vi "SeCrTs-UI Commands_R.vi"(9 "Er":refnum<queue>, 11 "Message Queue":refnum<queue>) -> ()   [LabVIEW 2022 SP3]
doc: "Use this template to build a simple state machine design pattern. Each state executes code and determines which state to transition to."
uses:
  RT Controls/SeCrTs-Message Cluster_R.ctl
  RT Controls/SeCrTs-NS Enum.ctl
  RT Controls/SeCrTs-Data Type Control screen.ctl
  RT Support/SeCrTs-RT_Global_R.vi
  <resource>/objmgr/ni.dex.rc
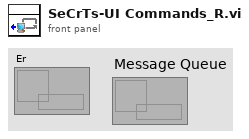
[diagram p1: front panel]
types:
  T1 = typedef "SeCrTs-NS Enum.ctl" = enum16{"Initialize", "Listen for UI Writer", "Receive UI Commands"}
  T2 = typedef "SeCrTs-Data Type Control screen.ctl" = cluster{"DI_Data":digitalwaveform[], "Drive_A_C":waveform(dbl)[], "Drive_A_D":waveform(dbl)[], "Drive_L_C":waveform(dbl)[], "Drive_L_D":waveform(dbl)[], "Loop Status":bool[], "CDT Timer":dbl, "RT Error":cluster{"Error Code":string, "Error Source":string}, "DO":waveform(dbl)[], "SEQ Monitor":string[]}
  T3 = typedef "SeCrTs-Message Cluster_R.ctl" = cluster{"Message":string, "Message Data":variant}
  T4 = typedef "Message Cluster_R.ctl" = cluster{"Message":string, "Message Data":variant}
  T5 = cluster{"Start DAQ":bool, "Stop DAQ":bool, "RT Stop":bool, "RT Exit":bool, "Start Seq":bool}
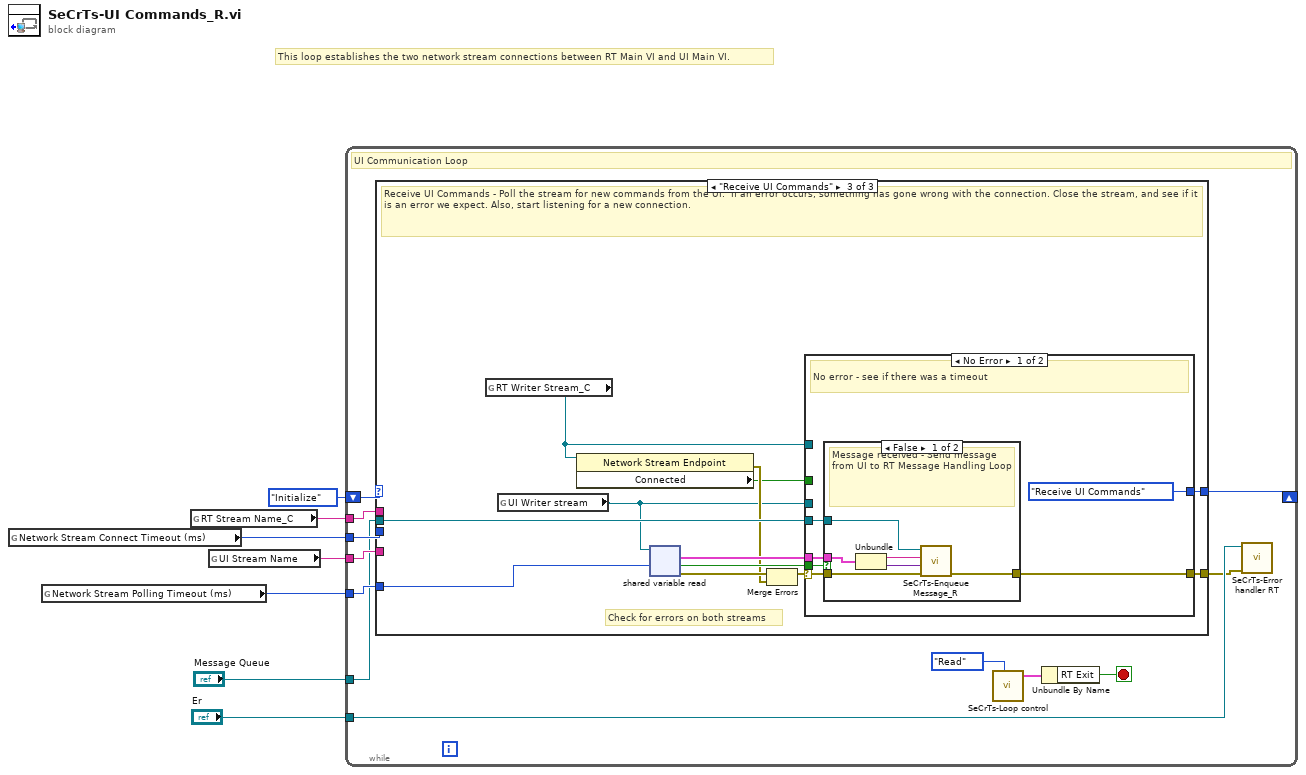
[diagram p0: block diagram]
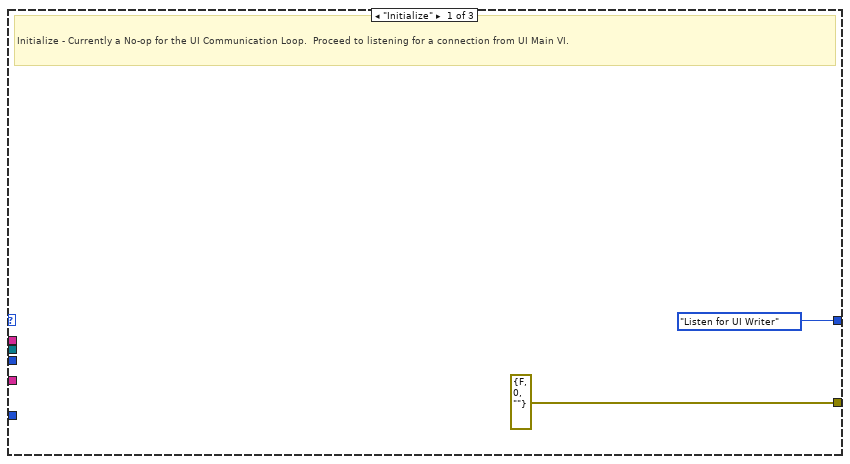
[diagram p2: hidden frame]
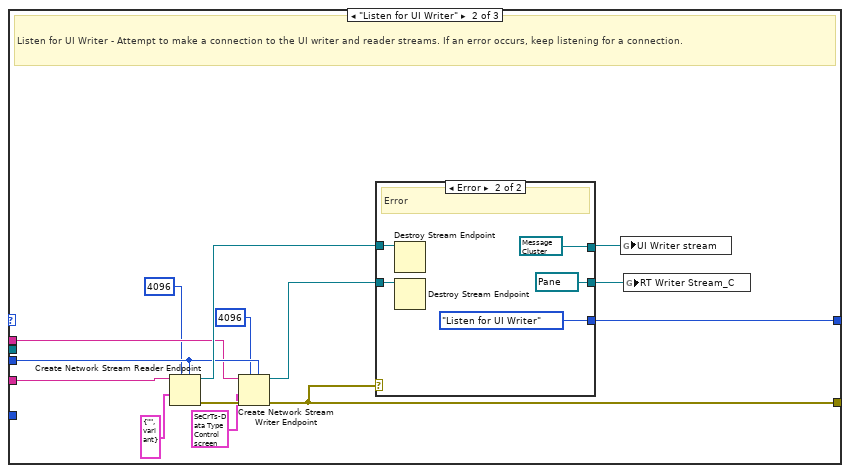
[diagram p3: hidden frame]
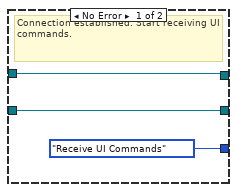
[diagram p4: hidden frame]
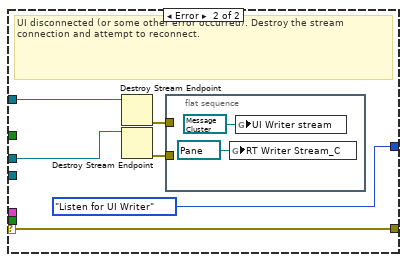
[diagram p6: hidden frame]
diagram:
  # "This loop establishes the two network stream connections between RT Main VI and UI Main VI."
  n1 = global read "SeCrTs-RT_Global_R.vi" "Network Stream Connect Timeout (ms)"() -> (w7:i32)
  n2 = global read "SeCrTs-RT_Global_R.vi" "Network Stream Polling Timeout (ms)"() -> (w6:i32)
  n3 = global read "SeCrTs-RT_Global_R.vi" "RT Stream Name_C"() -> (w3:string)
  n4 = global read "SeCrTs-RT_Global_R.vi" "UI Stream Name"() -> (w2:string)
  n5 = while {
    tunnel: "Message Queue" -> [w13]
    tunnel: w2 -> [w19]
    tunnel: w3 -> [w18]
    tunnel: w6 -> [w17]
    tunnel: w7 -> [w16]
    shift-right: [w14] -> _
    shift-left: SeCrTs-NS_Enum."Initialize" ("Enum") -> [w15]
    tunnel: "Er" -> [w9]
    stop <- w10 stop-if-true
    # "UI Communication Loop"
    n6 = case shown="\"Receive UI Commands\"" w15 {
      tunnel: [errorcluster {"status"=FALSE, "code"=0, "source"=""} ("error IO") w31 w55] -> w8
      tunnel: w16 -> [_ w30 _]
      tunnel: w19 -> [_ w34 _]
      tunnel: w13 -> [_ _ w54]
      tunnel: w18 -> [_ w29 _]
      tunnel: w17 -> [_ _ w47]
      tunnel: [SeCrTs-NS_Enum."Listen for UI Writer" ("Enum") w26 w44] -> w14
      frame "Initialize" {
        # "Initialize - Currently a No-op for the UI Communication Loop.  Proceed to listening for a connection from UI Main VI."
      }
      frame "Listen for UI Writer" {
        # "Listen for UI Writer - Attempt to make a connection to the UI writer and reader streams. If an error occurs, keep listening for a connection."
        n7 = Create Network Stream Reader Endpoint(5:w30, 7:4096 ("reader buffer size"), 9:T3 {"Message"="", "Message Data"=variant} ("Message Cluster"), 11:w34) -> (0:w33:errorcluster, 3:w35:refnum<k21>)  [unwired: 3 in]
        n8 = Create Network Stream Writer Endpoint(5:w30, 7:4096 ("writer buffer size"), 8:w33, 9:T2 {"DI_Data"=[], "Drive_A_C"=[], "Drive_A_D"=[], "Drive_L_C"=[], "Drive_L_D"=[], "Loop Status"=[], "CDT Timer"=0.0, "RT Error"={"Error Code"="", "Error Source"=""}, "DO"=[], "SEQ Monitor"=[]}, 11:w29) -> (0:w31:errorcluster, 3:w32:refnum<k21>)  [unwired: 2 in]
        n9 = case shown="Error" w31 {
          tunnel: w35 -> [w38 w43]
          tunnel: w32 -> [w36 w42]
          tunnel: [w38 refnum<k21> refnum ("reader endpoint")] -> w25
          tunnel: [SeCrTs-NS_Enum."Receive UI Commands" ("Enum") SeCrTs-NS_Enum."Listen for UI Writer" ("Enum")] -> w26
          tunnel: [w36 refnum<k21> refnum ("RT Stream Name_C")] -> w22
          frame No Error {
            # "Connection established. Start receiving UI commands."
          }
          frame Error {
            # "Error"
            n10 = Destroy Stream Endpoint(11:w43) -> ()  [unwired: 1 in, 1 out]
            n11 = Destroy Stream Endpoint(11:w42) -> ()  [unwired: 1 in, 1 out]
          }
        }
        n12 = global write "SeCrTs-RT_Global_R.vi" "UI Writer stream"(w25) -> ()
        n13 = global write "SeCrTs-RT_Global_R.vi" "RT Writer Stream_C"(w22) -> ()
      }
      frame "Receive UI Commands" {
        # "Check for errors on both streams"
        # "Receive UI Commands - Poll the stream for new commands from the UI.  If an error occurs, something has gone wrong with the connection. Close the stream, and see if it is an error we expect. Also, start listening for a new connection."
        n14 = global read "SeCrTs-RT_Global_R.vi" "RT Writer Stream_C"() -> (w46:refnum<k21>)
        n15 = global read "SeCrTs-RT_Global_R.vi" "UI Writer stream"() -> (w45:refnum<k21>)
        n16 = property class="Network Stream Endpoint"(reference=w46) -> (error out=w49:errorcluster, "Connected"=w48:bool)  [unwired: 1 in, 1 out]
        n17 = shared-variable-read(w45, w47) -> (w51:errorcluster, w52:bool, w53:T4)  [unwired: 1 in, 1 out]
        n18 = Merge Errors(w51, w49) -> (w50:errorcluster)
        n19 = case shown="No Error" w50 {
          selector: w50 -> [w59 w74]
          tunnel: [w58 w74] -> w55
          tunnel: w52 -> [w61 _]
          tunnel: w53 -> [w60 _]
          tunnel: [SeCrTs-NS_Enum."Receive UI Commands" ("Enum") SeCrTs-NS_Enum."Listen for UI Writer" ("Enum")] -> w44
          tunnel: w54 -> [w57 _]
          tunnel: w45 -> [_ w71]
          tunnel: w48 -> [_ _]
          tunnel: w46 -> [_ w70]
          frame No Error {
            # "No error - see if there was a timeout"
            n20 = case shown="False" w61 {
              tunnel: w60 -> [w67 _]
              tunnel: w59 -> [w65 w68]
              tunnel: [w66 w68] -> w58
              tunnel: w57 -> [w64 _]
              frame False {
                # "Message received - Send message from UI to RT Message Handling Loop"
                n21 = Unbundle(w67) -> ("Message"=w63:string, "Message Data"=w62:variant)
                n22 = call "SeCrTs-Enqueue Message_R.vi"("error in (no error)"=w65, "Message Data"=w62, "Message"=w63, "Message Queue"=w64) -> ("error out"=w66:errorcluster)  [unwired: 6 in, 1 out]
              }
              frame True {
                # "Timeout - no new command"
              }
            }
          }
          frame Error {
            # "UI disconnected (or some other error occurred). Destroy the stream connection and attempt to reconnect."
            n23 = Destroy Stream Endpoint(11:w70) -> (0:w73:errorcluster)  [unwired: 1 in]
            n24 = Destroy Stream Endpoint(11:w71) -> (0:w72:errorcluster)  [unwired: 1 in]
            n25 = flat-sequence {
              tunnel: w73 -> [_]
              tunnel: w72 -> [_]
              frame #0 {
                n26 = global write "SeCrTs-RT_Global_R.vi" "RT Writer Stream_C"(refnum<k21> refnum ("RT Writer Stream_C")) -> ()
                n27 = global write "SeCrTs-RT_Global_R.vi" "UI Writer stream"(refnum<k21> refnum ("UI Writer stream")) -> ()
              }
            }
          }
        }
      }
    }
    n28 = call "SeCrTs-Loop control.vi"("Action"=enum16{"Init", "Write", "Read"}."Read") -> ("Loop Control out"=w11:T5)  [unwired: 9 in, 1 out]
    n29 = Unbundle By Name(w11) -> ("RT Exit"=w10:bool)
    n30 = call "SeCrTs-Error handler RT.vi"("error in"=w8, "Message Queue"=w9) -> ()  [unwired: 8 in, 2 out]
  }
